vi "main(test).vi"() -> ()   [LabVIEW 2020]
uses:
  stany.ctl
  <vilib>/Analysis/1siggen.llb/Ramp Pattern by Samples.vi
  <vilib>/Utility/file.llb/Write Delimited Spreadsheet (DBL).vi
  lib/VirtualLab.lvlibp/VISASimulator/VISALib.lvlib
  lib/VirtualLab.lvlibp/Devices/Devices.lvlib
  lib/VirtualLab.lvlibp/Models/Exercise.lvlib
  <vilib>/Analysis/NI_AALBase.lvlib
panel:
  in  "Samples":i32=800
  out "Error":bool
  out "Error source":string
  in  "Save":bool
  out "Connection HP_dvm1":bool
  out "Actual Power [mW]":dbl
  in  "Pmax [mW]":dbl=200.0
  in  "Ib[uA]":dbl(ring) items=["0"=0.0, "100"=0.0001, "200"=0.0002, "300"=0.0003, "400"=0.0004]
  out "Ic=f(Uce)":cluster{dbl[], "Ramp Pattern":dbl[]}(graph)
  out "Ic[A]":dbl
  out "Uce [V]":dbl
  in  "Cancel Button":bool
  out "Progres":u8(slide) scale=0.0..100.0
  in  "stop/resume":bool
  in  "Measure":bool
  in  "Connect":bool
  out "Connection HP_zas":bool
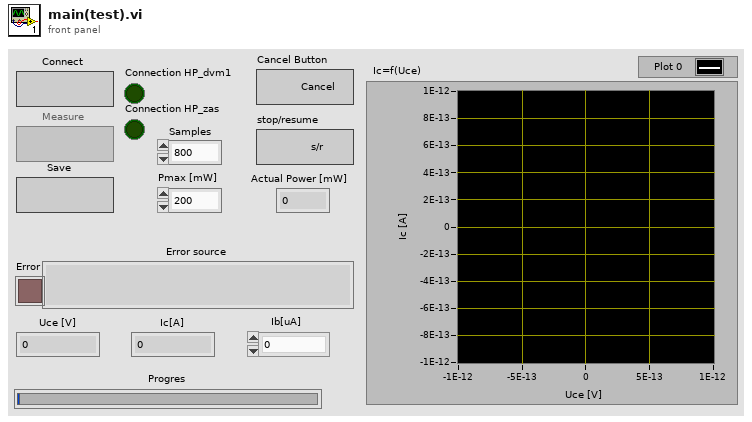
[diagram p1: front panel]
types:
  T1 = cluster{"HP_zas (PSU reference)":refnum<visa-resource-name>, "PSU_connecton":bool, "Ic":dbl[], "Uce":dbl[], "HP_dvm1(DMM reference)":refnum<visa-resource-name>, "DMM_connecton":bool}
  T2 = typedef "stany.ctl" = enum16{"init", "wait", "connect", "measure", "end", "save", "error"}
  T3 = enum8{"Enabled", "Disabled", "Disabled and Grayed Out"}
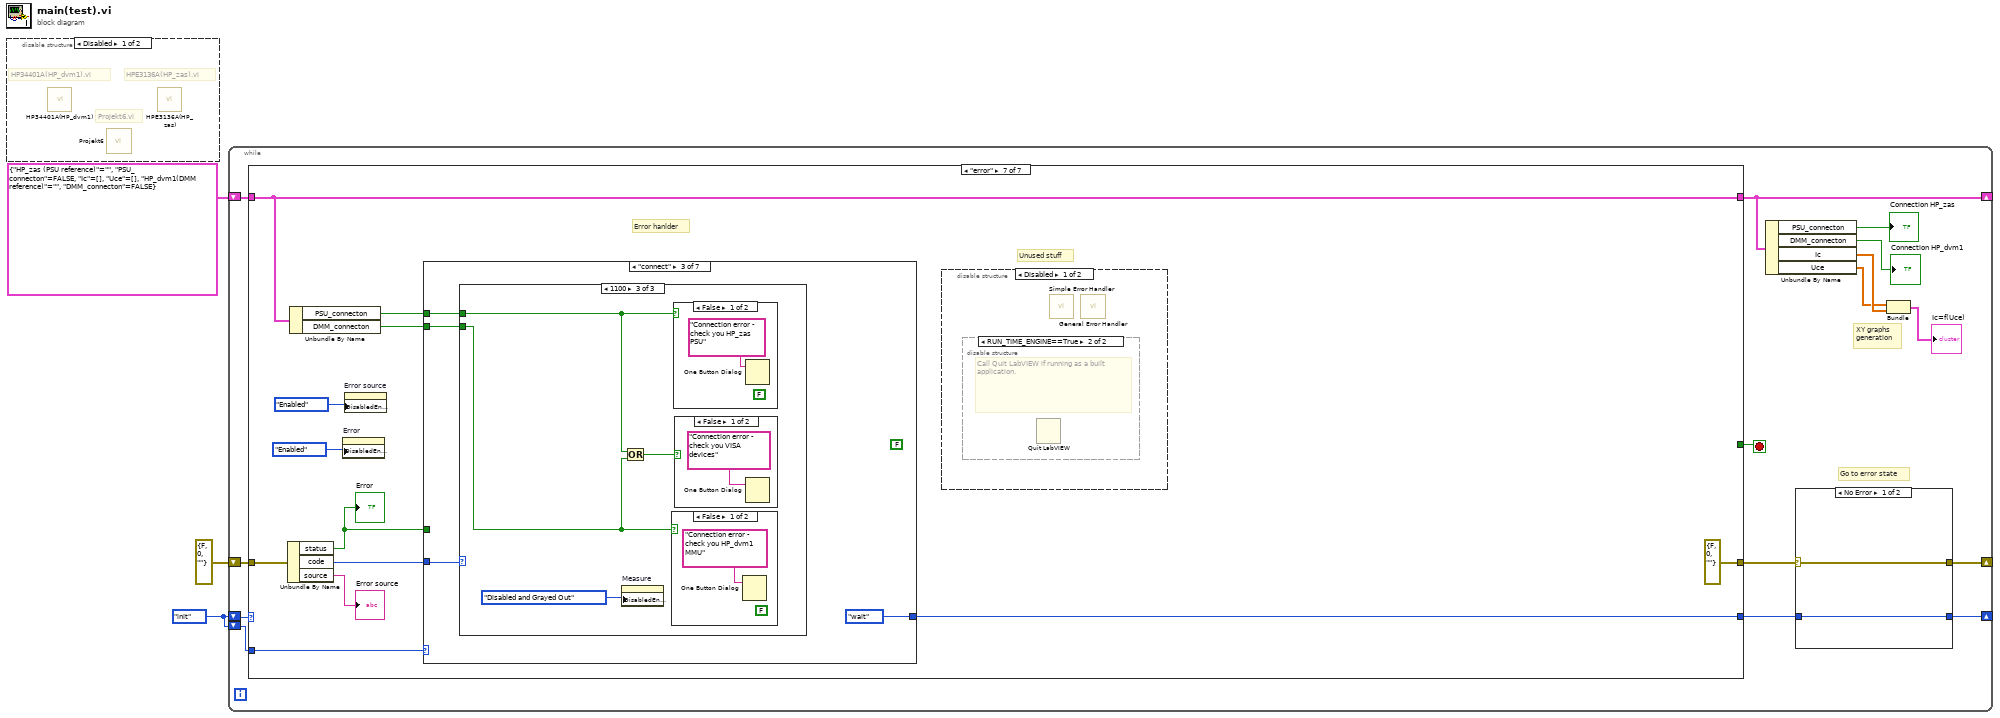
[diagram p0: block diagram]
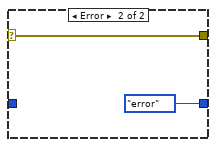
[diagram p3: hidden frame]
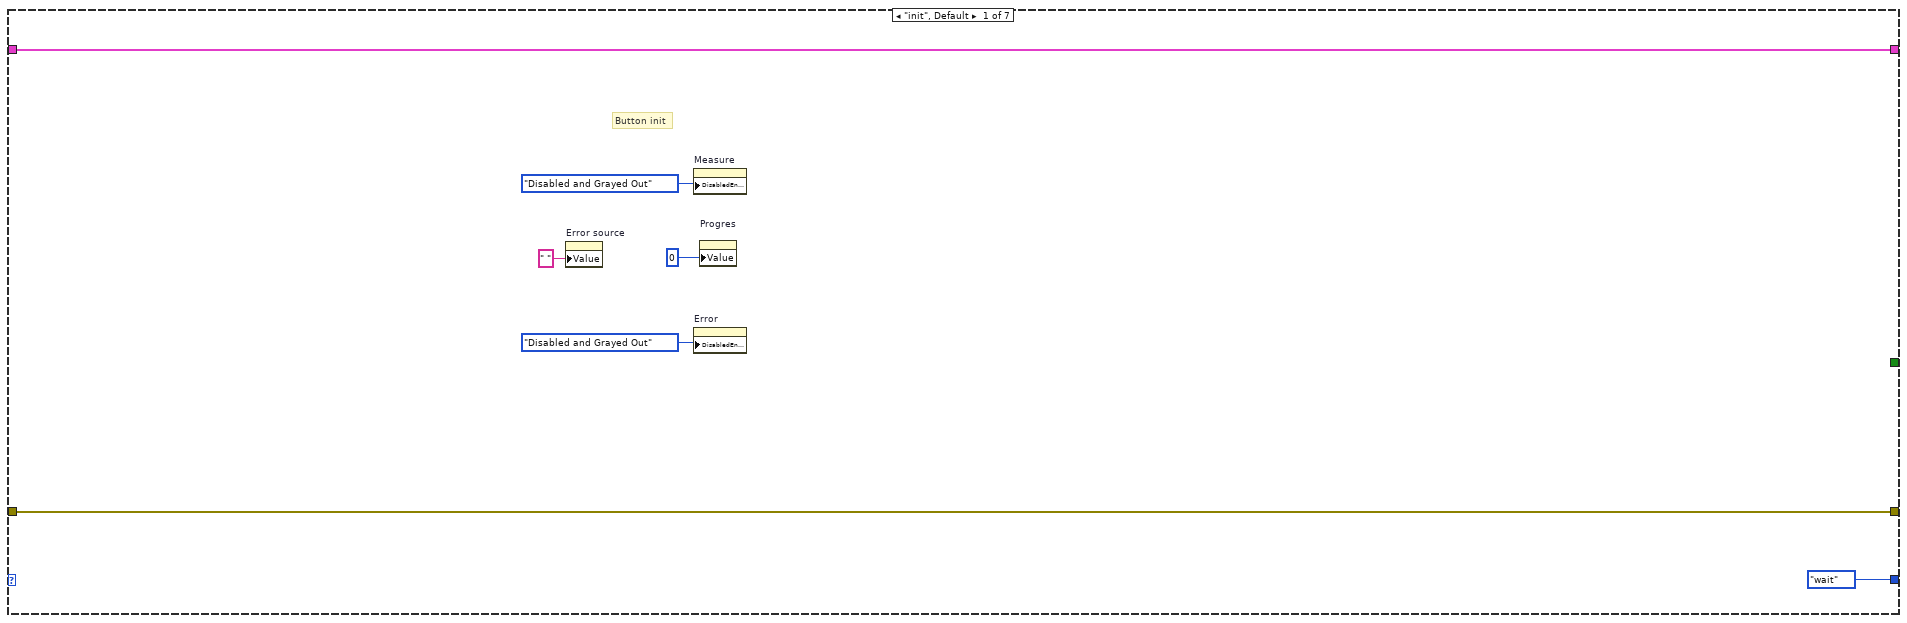
[diagram p4: hidden frame]
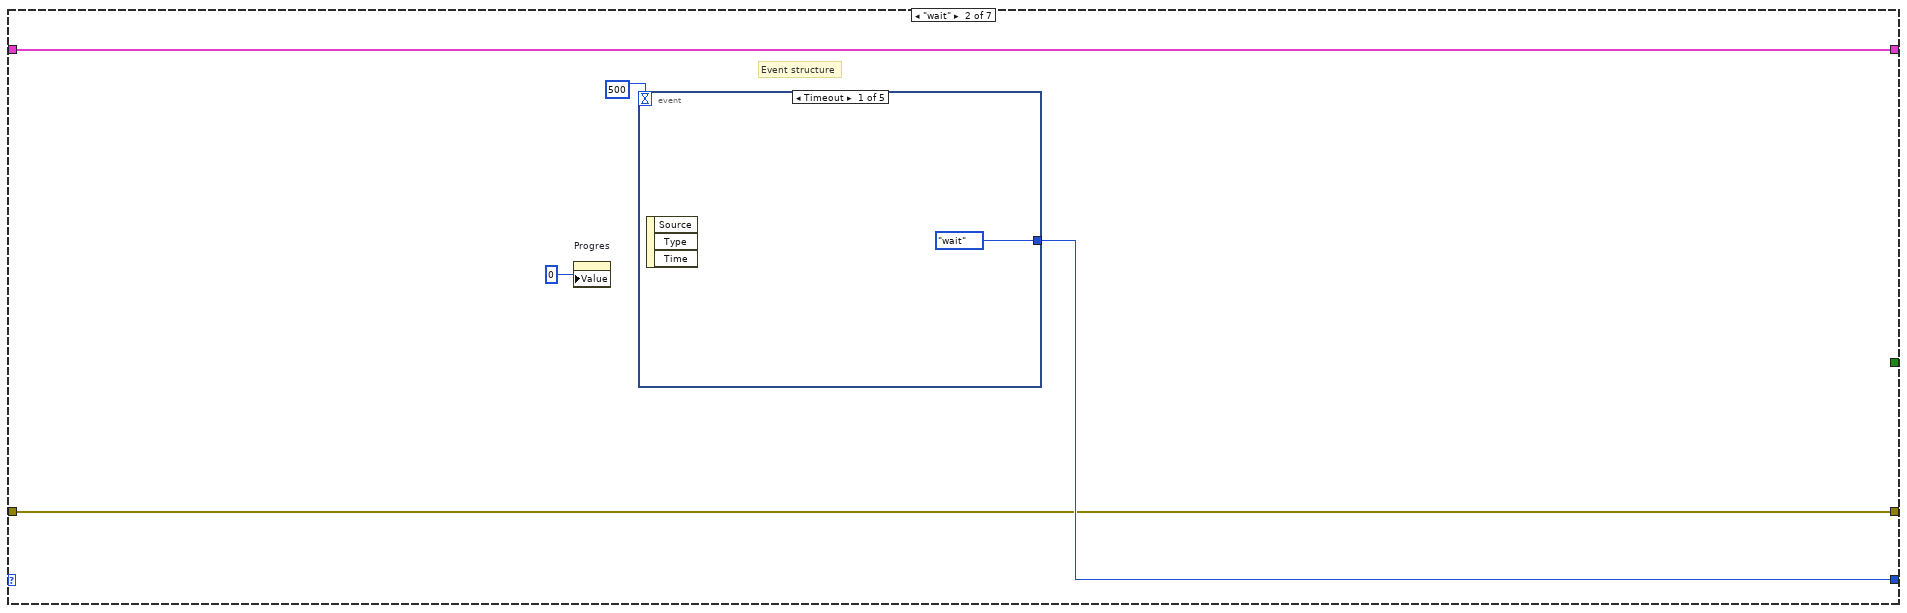
[diagram p5: hidden frame]
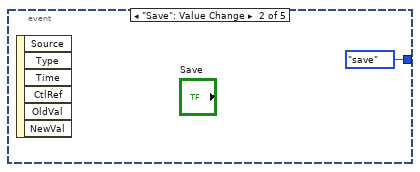
[diagram p6: hidden frame]
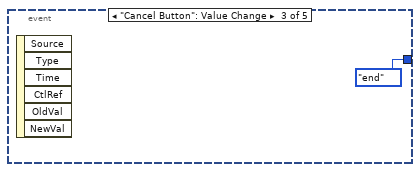
[diagram p7: hidden frame]
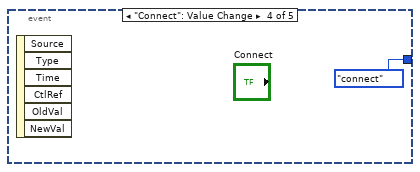
[diagram p8: hidden frame]
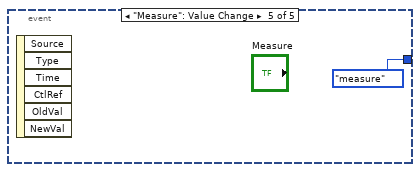
[diagram p9: hidden frame]
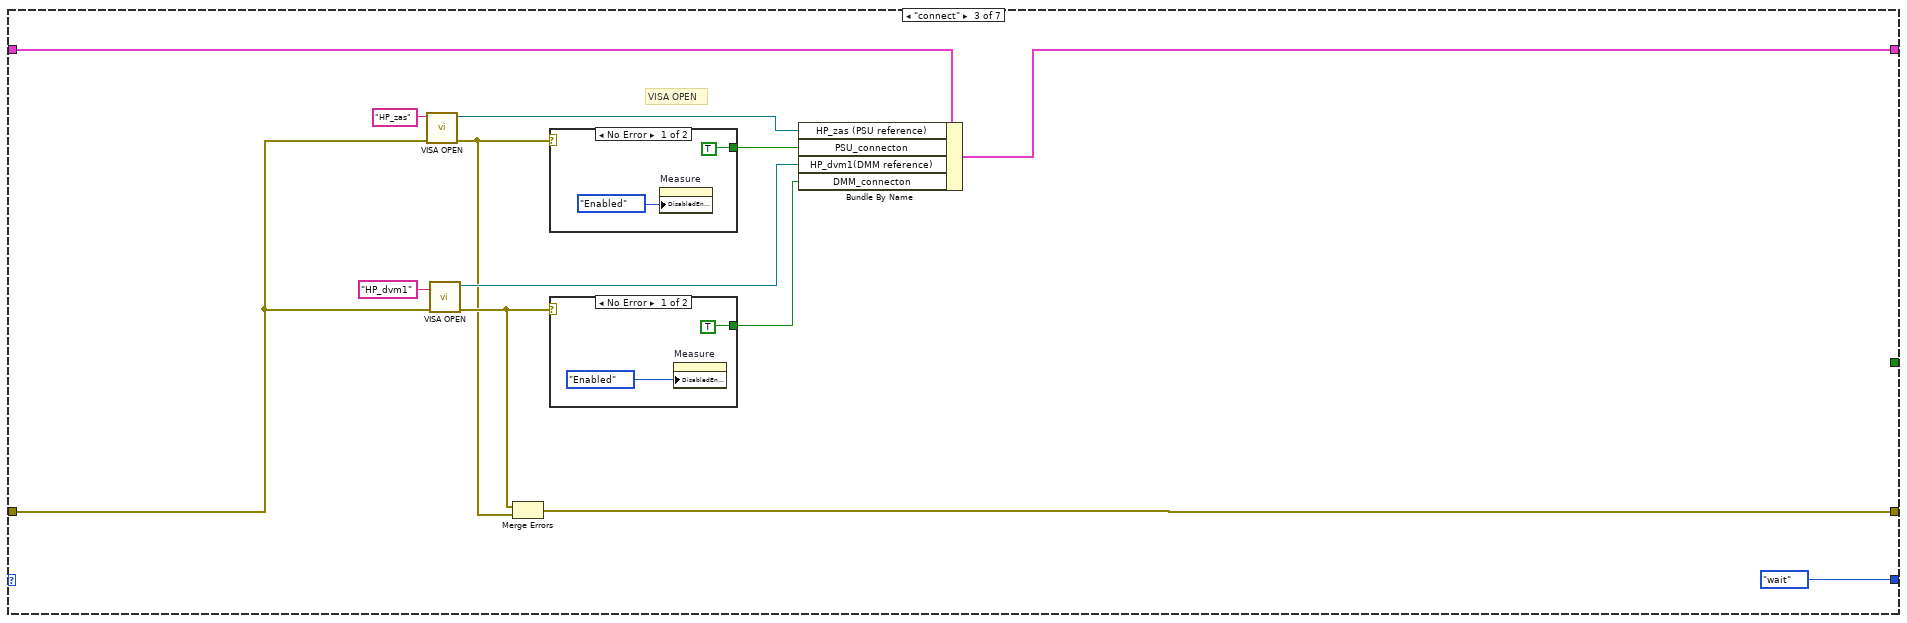
[diagram p10: hidden frame]
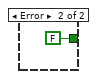
[diagram p11: hidden frame]
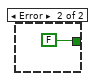
[diagram p12: hidden frame]
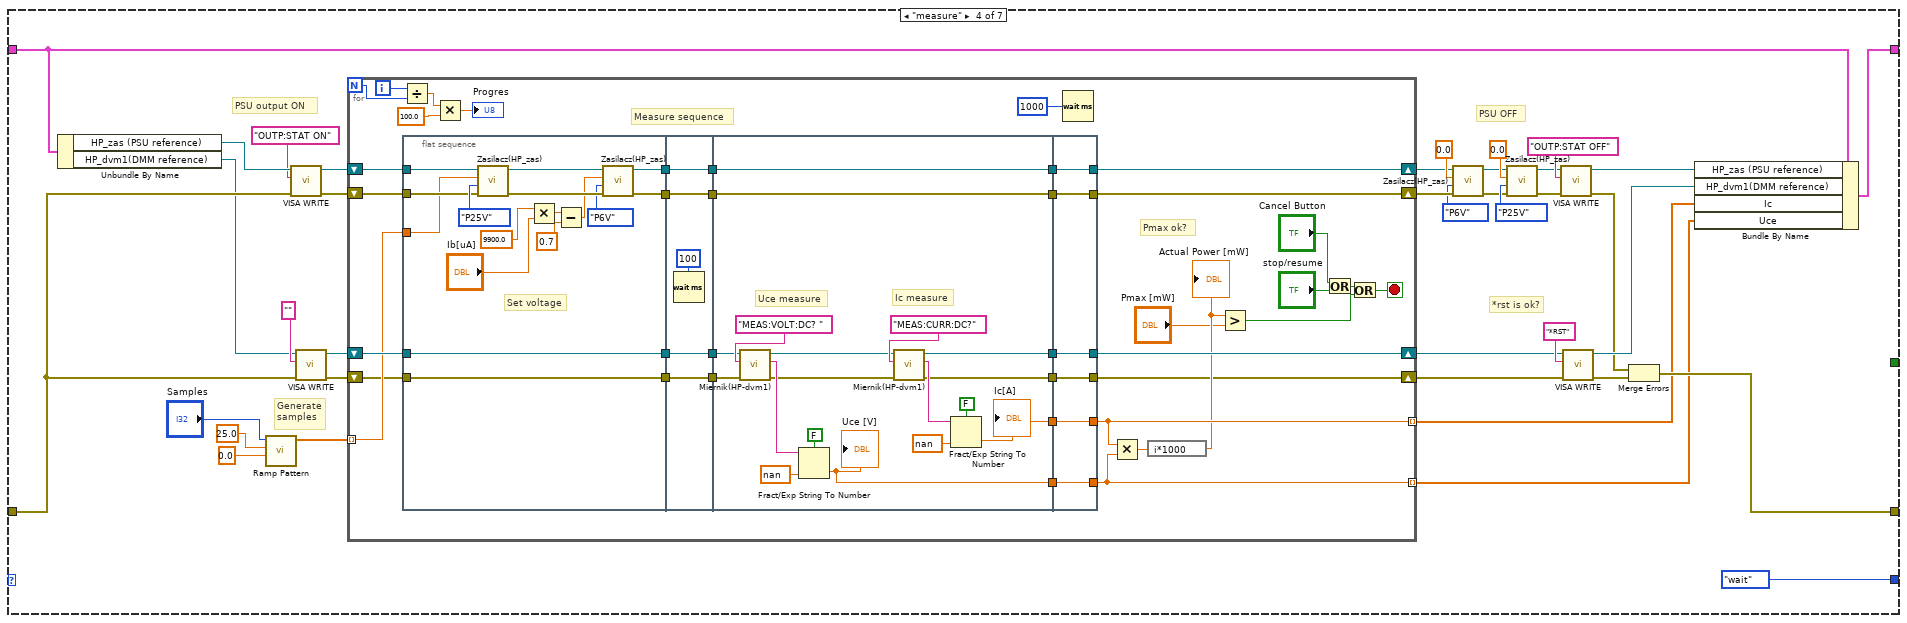
[diagram p13: hidden frame]
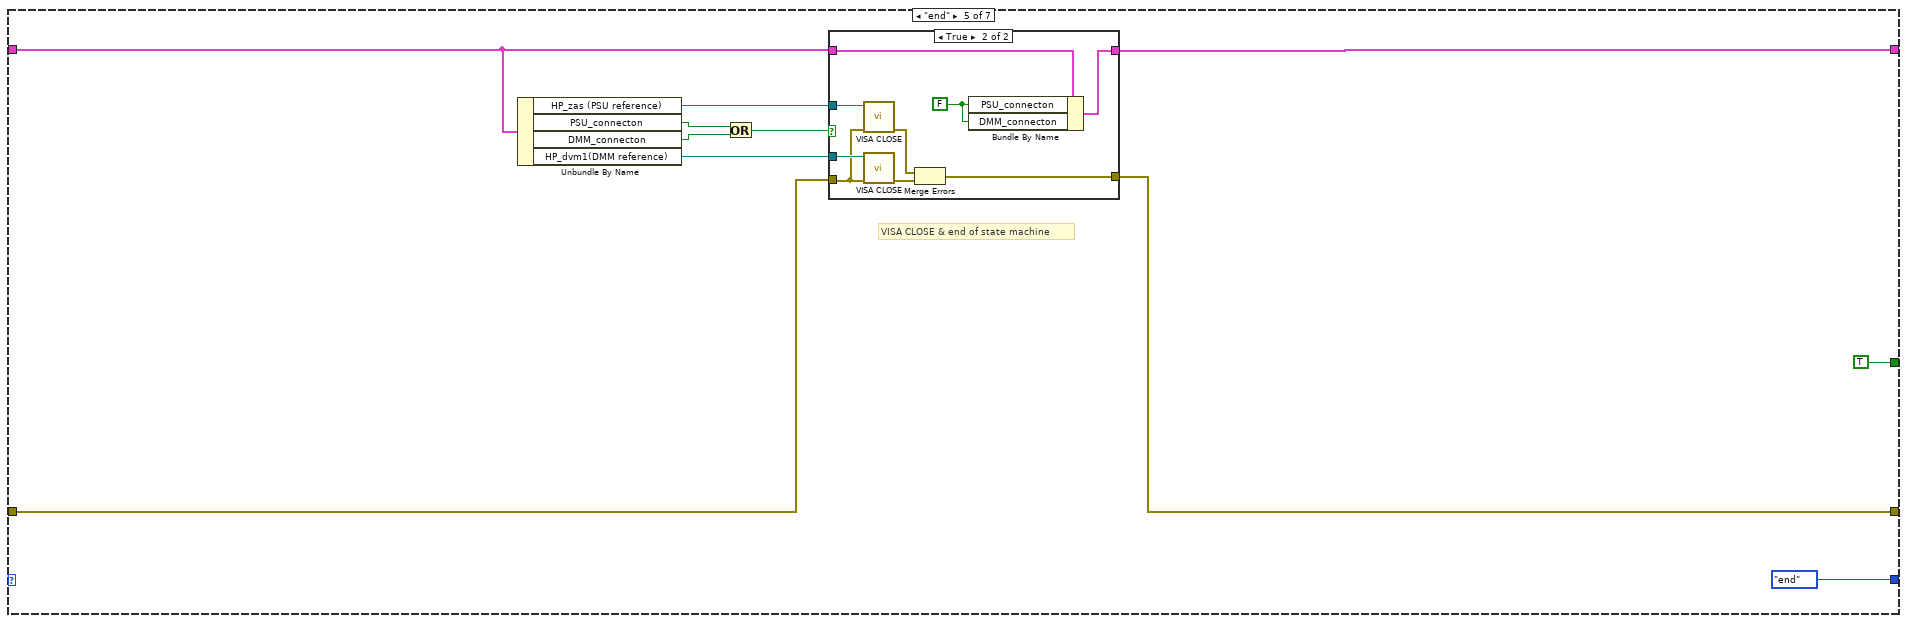
[diagram p14: hidden frame]
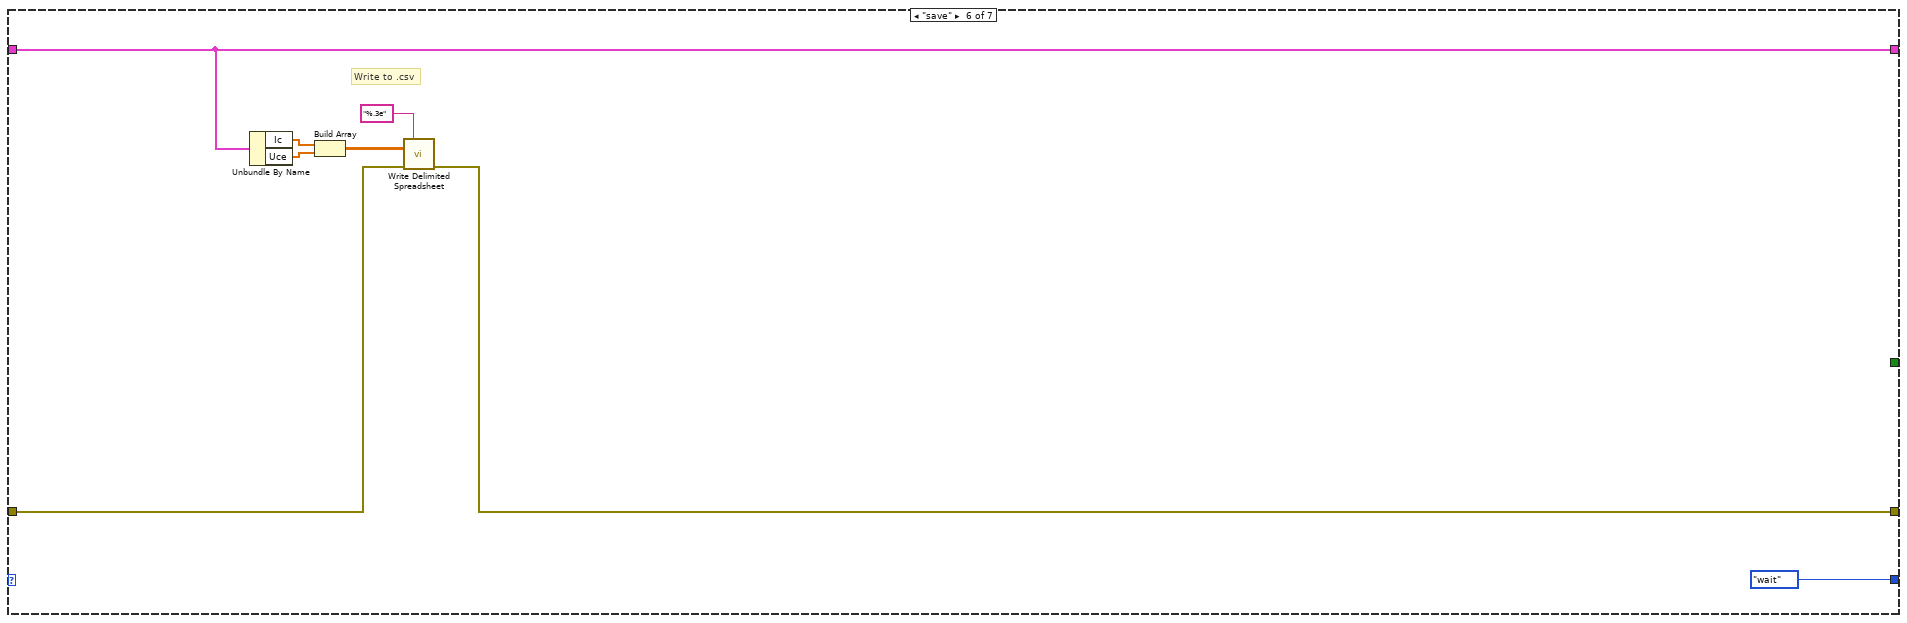
[diagram p16: hidden frame]
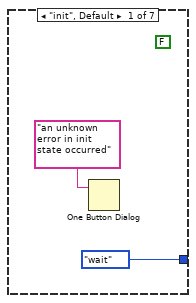
[diagram p19: hidden frame]
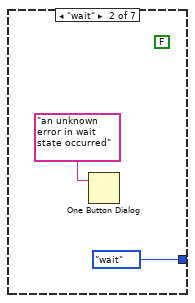
[diagram p20: hidden frame]
diagram:
  w1 = stany."init"
  n1 = disable-structure shown="Disabled" {
    frame Disabled {
      # "Projekt6.vi"
      # "HPE3136A(HP_zas).vi"
      # "HP34401A(HP_dvm1).vi"
      n2 = call "HP34401A(HP_dvm1).vi"() -> ()  [unwired: 12 in]
      n3 = call "Projekt6.vi"() -> ()  [unwired: 12 in]
      n4 = call "HPE3136A(HP_zas).vi"() -> ()  [unwired: 12 in]
    }
    frame Enabled {
    }
  }
  n5 = while {
    shift-right: [w10] -> _
    shift-left: w1 -> [w18]
    shift-right: [w9] -> _
    shift-left: T1 {"HP_zas (PSU reference)"="", "PSU_connecton"=FALSE, "Ic"=[], "Uce"=[], "HP_dvm1(DMM reference)"="", "DMM_connecton"=FALSE} -> [w16]
    shift-right: [w12] -> _
    shift-left: errorcluster {"status"=FALSE, "code"=0, "source"=""} ("error constant") -> [w14]
    shift-left: w1 -> [w7]
    stop <- w17 stop-if-true
    # "Go to error state"
    # "XY graphs\ngeneration"
    n6 = case shown="\"error\"" w18 {
      tunnel: [stany."wait" w33 stany."wait" stany."wait" stany."end" stany."wait" w215] -> w11
      tunnel: [_ _ _ _ TRUE _ _] -> w17
      tunnel: w16 -> [w27 w32 w46 w78 w186 w208 w212]
      tunnel: [w27 w32 w48 w94 w187 w208 w212] -> w9
      tunnel: w14 -> [w25 w30 w40 w76 w181 w202 w219]
      tunnel: [w25 w30 w43 w73 w180 w203 errorcluster {"status"=FALSE, "code"=0, "source"=""} ("error out")] -> w13
      tunnel: w7 -> [_ _ _ _ _ _ w220]
      frame "init", Default {
        # "Button init"
        n7 = property on="Error source" class="Str"("Value"=" " ("Error source")) -> ()  [unwired: 2 in, 2 out]
        n8 = property on="Measure" class="Bool"("DisabledEnum"=T3."Disabled and Grayed Out" ("Disabled")) -> ()  [unwired: 2 in, 2 out]
        n9 = property on="Error" class="Bool (strict)"("DisabledEnum"=T3."Disabled and Grayed Out" ("Disabled")) -> ()  [unwired: 2 in, 2 out]
        n10 = property on="Progres" class="Slide (strict)"("Value"=u8 0 ("Progres")) -> ()  [unwired: 2 in, 2 out]
      }
      frame "wait" {
        # "Event structure"
        n11 = property on="Progres" class="Slide (strict)"("Value"=u8 0 ("Progres")) -> ()  [unwired: 2 in, 2 out]
        n12 = event shown="[0] Timeout" {
          selector: _ -> [_ _ _ _ _]
          dyn-events: _ -> [_ _ _ _ _]
          timeout: 500 -> [_ _ _ _ _]
          tunnel: [stany."wait" stany."save" stany."end" stany."connect" stany."measure"] -> w33
          event Timeout {
            n13 = event-data() -> ()  [unwired: 1 in, 3 out]
          }
          event "Save": Value Change {
            n14 = event-data() -> ()  [unwired: 1 in, 6 out]
          }
          event "Cancel Button": Value Change {
            n15 = event-data() -> ()  [unwired: 1 in, 6 out]
          }
          event "Connect": Value Change {
            n16 = event-data() -> ()  [unwired: 1 in, 6 out]
          }
          event "Measure": Value Change {
            n17 = event-data() -> ()  [unwired: 1 in, 6 out]
          }
        }
      }
      frame "connect" {
        # "VISA OPEN"
        n18 = call "VISA OPEN.vi"("error in (no error)"=w40, "VISA resource name"="HP_zas") -> ("error out"=w41:errorcluster, "VISA resource name out"=w51:refnum<visa-resource-name>)  [unwired: 8 in]
        n19 = call "VISA OPEN.vi"("error in (no error)"=w40, "VISA resource name"="HP_dvm1") -> ("error out"=w42:errorcluster, "VISA resource name out"=w45:refnum<visa-resource-name>)  [unwired: 8 in]
        n20 = Merge Errors(w42, w41) -> (w43:errorcluster)
        n21 = case shown="No Error" w41 {
          tunnel: [TRUE FALSE ("connecton")] -> w50
          frame No Error {
            n22 = property on="Measure" class="Bool"("DisabledEnum"=T3."Enabled" ("Disabled")) -> ()  [unwired: 2 in, 2 out]
          }
          frame Error {
          }
        }
        n23 = case shown="No Error" w42 {
          tunnel: [TRUE FALSE ("connecton")] -> w44
          frame No Error {
            n24 = property on="Measure" class="Bool"("DisabledEnum"=T3."Enabled" ("Disabled")) -> ()  [unwired: 2 in, 2 out]
          }
          frame Error {
          }
        }
        n25 = Bundle By Name(cluster=w46, "HP_zas (PSU reference)"=w51, "PSU_connecton"=w50, "HP_dvm1(DMM reference)"=w45, "DMM_connecton"=w44) -> (w48:T1)
      }
      frame "measure" {
        # "PSU output ON"
        # "Generate\nsamples"
        # "*rst is ok?"
        # "PSU OFF"
        n26 = Unbundle By Name(w78) -> ("HP_zas (PSU reference)"=w70:refnum<visa-resource-name>, "HP_dvm1(DMM reference)"=w59:refnum<visa-resource-name>)
        n27 = call-poly <vilib>:"Ramp Pattern.vi"("start"=0.0, "end"=25.0, "samples"="Samples") -> ("Ramp Pattern"=w63:dbl[])  [unwired: 7 in, 1 out]
        n28 = call "VISA WRITE.vi"("error in (no error)"=w76, "write buffer"="OUTP:STAT ON" ("format string"), "VISA resource name"=w70) -> ("error out"=w64:errorcluster, "VISA resource name out"=w67:refnum<visa-resource-name>)  [unwired: 6 in, 1 out]
        n29 = call "VISA WRITE.vi"("error in (no error)"=w76, "write buffer"="" ("format string"), "VISA resource name"=w59) -> ("error out"=w61:errorcluster, "VISA resource name out"=w62:refnum<visa-resource-name>)  [unwired: 6 in, 1 out]
        n30 = for {
          N -> [w127]
          shift-right: [w123] -> w84
          shift-left: w67 -> [w115]
          tunnel: [w107] -> w71 mode=indexing
          shift-right: [w122] -> w83
          shift-left: w64 -> [w114]
          tunnel: w63 -> [w110] mode=indexing
          tunnel: [w108] -> w72 mode=indexing
          shift-right: [w120] -> w80
          shift-left: w62 -> [w111]
          shift-right: [w100] -> w79
          shift-left: w61 -> [w98]
          i -> [w128]
          stop <- w101 stop-if-true
          # "Pmax ok?"
          # "Measure sequence"
          n31 = Divide(x=w128, y=w127) -> (x/y=w133:dbl)
          n32 = flat-sequence {
            tunnel: [w143] -> w118
            tunnel: [w144] -> w116
            tunnel: w115 -> [w149]
            tunnel: w114 -> [w148]
            tunnel: [w147] -> w112
            tunnel: w111 -> [w147]
            tunnel: w110 -> [w141]
            tunnel: w98 -> [w135]
            tunnel: [w135] -> w97
            tunnel: [w154] -> w119
            tunnel: w118 -> [w154]
            tunnel: [w153] -> w117
            tunnel: w116 -> [w153]
            tunnel: [w152] -> w113
            tunnel: w112 -> [w152]
            tunnel: w97 -> [w151]
            tunnel: [w151] -> w96
            tunnel: [w167] -> w126
            tunnel: [w168] -> w125
            tunnel: [w169] -> w124
            tunnel: [w159] -> w121
            tunnel: w119 -> [w168]
            tunnel: w117 -> [w167]
            tunnel: w113 -> [w166]
            tunnel: [w158] -> w109
            tunnel: [w157] -> w99
            tunnel: w96 -> [w156]
            tunnel: w126 -> [w178]
            tunnel: w125 -> [w177]
            tunnel: w124 -> [w179]
            tunnel: [w179] -> w107
            tunnel: [w178] -> w123
            tunnel: [w177] -> w122
            tunnel: w121 -> [w176]
            tunnel: [w176] -> w120
            tunnel: w109 -> [w175]
            tunnel: [w175] -> w108
            tunnel: [w174] -> w100
            tunnel: w99 -> [w174]
            frame #0 {
              # "Set voltage"
              n33 = call "Zasilacz(HP_zas).vi"("error in (no error)"=w148, "Source"=enum16{"P6V", "P25V"}."P25V" ("Kanal"), "Voltage"=w141, "VISA Refnum in"=w149) -> ("error out"=w145:errorcluster, "VISA Refnum out"=w146:refnum<visa-resource-name>)  [unwired: 6 in]
              n34 = Multiply(x=9900.0, y="Ib[uA]") -> (x*y=w138:dbl)
              n35 = Subtract(x=w138, y=0.7) -> (x-y=w140:dbl)
              n36 = call "Zasilacz(HP_zas).vi"("error in (no error)"=w145, "Source"=enum16{"P6V", "P25V"}."P6V" ("Kanal"), "Voltage"=w140, "VISA Refnum in"=w146) -> ("error out"=w143:errorcluster, "VISA Refnum out"=w144:refnum<visa-resource-name>)  [unwired: 6 in]
            }
            frame #1 {
              n37 = Wait (ms)(milliseconds to wait=u32 100) -> ()  [unwired: 1 out]
            }
            frame #2 {
              # "Ic measure"
              # "Uce measure"
              n38 = call "Miernik(HP-dvm1).vi"("error in (no error)"=w156, "write buffer"="MEAS:VOLT:DC? ", "VISA Refnum in"=w166) -> ("error out"=w161:errorcluster, "read buffer"=w173:string, "VISA Refnum out"=w160:refnum<visa-resource-name>)  [unwired: 6 in]
              n39 = Fract/Exp String To Number(use system decimal point (T)=FALSE, string=w173, default (0 dbl)=nan) -> (number=w169:dbl)  [unwired: 1 in, 1 out]
              "Uce [V]" <- w169
              n40 = call "Miernik(HP-dvm1).vi"("error in (no error)"=w161, "write buffer"="MEAS:CURR:DC?", "VISA Refnum in"=w160) -> ("error out"=w157:errorcluster, "read buffer"=w165:string, "VISA Refnum out"=w159:refnum<visa-resource-name>)  [unwired: 6 in]
              n41 = Fract/Exp String To Number(use system decimal point (T)=FALSE, string=w165, default (0 dbl)=nan) -> (number=w158:dbl)  [unwired: 1 in, 1 out]
              "Ic[A]" <- w158
            }
            frame #3 {
            }
          }
          n42 = Multiply(x=w133, y=100.0) -> (x*y=→"Progres":dbl)
          n43 = Wait (ms)(milliseconds to wait=u32 1000) -> ()  [unwired: 1 out]
          n44 = Multiply(x=w108, y=w107) -> (x*y=w106:dbl)
          n45 = expression code="i*1000"(w106) -> (w105:dbl)
          "Actual Power [mW]" <- w105
          n46 = Greater?(x=w105, y="Pmax [mW]") -> (0:w102:bool)
          n47 = Or(x="Cancel Button", y="stop/resume") -> (x .or. y?=w103:bool)
          n48 = Or(x=w103, y=w102) -> (x .or. y?=w101:bool)
        }
        n49 = call "Zasilacz(HP_zas).vi"("error in (no error)"=w83, "Source"=enum16{"P6V", "P25V"}."P6V" ("Kanal"), "Voltage"=0.0 ("Napiecie 2"), "VISA Refnum in"=w84) -> ("error out"=w86:errorcluster, "VISA Refnum out"=w85:refnum<visa-resource-name>)  [unwired: 6 in]
        n50 = call "Zasilacz(HP_zas).vi"("error in (no error)"=w86, "Source"=enum16{"P6V", "P25V"}."P25V" ("Kanal"), "Voltage"=0.0 ("Napiecie 2"), "VISA Refnum in"=w85) -> ("error out"=w88:errorcluster, "VISA Refnum out"=w89:refnum<visa-resource-name>)  [unwired: 6 in]
        n51 = call "VISA WRITE.vi"("error in (no error)"=w88, "write buffer"="OUTP:STAT OFF" ("format string"), "VISA resource name"=w89) -> ("error out"=w75:errorcluster, "VISA resource name out"=w93:refnum<visa-resource-name>)  [unwired: 6 in, 1 out]
        n52 = call "VISA WRITE.vi"("error in (no error)"=w79, "write buffer"="*RST" ("format string"), "VISA resource name"=w80) -> ("error out"=w74:errorcluster, "VISA resource name out"=w77:refnum<visa-resource-name>)  [unwired: 6 in, 1 out]
        n53 = Merge Errors(w75, w74) -> (w73:errorcluster)
        n54 = Bundle By Name(cluster=w78, "HP_zas (PSU reference)"=w93, "HP_dvm1(DMM reference)"=w77, "Ic"=w72, "Uce"=w71) -> (w94:T1)
      }
      frame "end" {
        # "VISA CLOSE & end of state machine"
        n55 = Unbundle By Name(w186) -> ("HP_zas (PSU reference)"=w188:refnum<visa-resource-name>, "PSU_connecton"=w184:bool, "DMM_connecton"=w183:bool, "HP_dvm1(DMM reference)"=w185:refnum<visa-resource-name>)
        n56 = Or(x=w184, y=w183) -> (x .or. y?=w182:bool)
        n57 = case shown="True" w182 {
          tunnel: w188 -> [_ w201]
          tunnel: w186 -> [w192 w200]
          tunnel: [w192 w198] -> w187
          tunnel: w185 -> [_ w197]
          tunnel: [w191 w194] -> w180
          tunnel: w181 -> [w191 w195]
          frame False {
          }
          frame True {
            w199 = FALSE ("connecton")
            n58 = call "VISA CLOSE.vi"("error in (no error)"=w195, "VISA resource name"=w201) -> ("error out"=w193:errorcluster)  [unwired: 9 in]
            n59 = call "VISA CLOSE.vi"("error in (no error)"=w195, "VISA resource name"=w197) -> ("error out"=w196:errorcluster)  [unwired: 9 in]
            n60 = Merge Errors(w193, w196) -> (w194:errorcluster)
            n61 = Bundle By Name(cluster=w200, "PSU_connecton"=w199, "DMM_connecton"=w199) -> (w198:T1)
          }
        }
      }
      frame "save" {
        # "Write to .csv"
        n62 = Unbundle By Name(w208) -> ("Ic"=w207:dbl[], "Uce"=w206:dbl[])
        n63 = Build Array(w207, w206) -> (w205:dbl[][])
        n64 = call-poly <vilib>:"Write Delimited Spreadsheet.vi"("format (%.3f)"="%.3e", "2D data"=w205, "error in (no error)"=w202) -> ("error out"=w203:errorcluster)  [unwired: 11 in, 1 out]
      }
      frame "error" {
        # "Unused stuff"
        # "Error hanlder"
        n65 = Unbundle By Name(w219) -> ("status"=w217:bool, "code"=w218:i32, "source"=→"Error source":string)
        "Error" <- w217
        n66 = Unbundle By Name(w212) -> ("PSU_connecton"=w211:bool, "DMM_connecton"=w210:bool)
        n67 = property on="Error" class="Bool (strict)"("DisabledEnum"=T3."Enabled" ("Disabled")) -> ()  [unwired: 2 in, 2 out]
        n68 = property on="Error source" class="Str"("DisabledEnum"=T3."Enabled" ("Disabled")) -> ()  [unwired: 2 in, 2 out]
        n69 = case shown="\"connect\"" w220 {
          tunnel: w218 -> [_ _ w229 _ _ _ _]
          tunnel: w217 -> [_ _ _ _ _ _ _]
          tunnel: [stany."wait" stany."wait" stany."wait" stany."wait" stany."wait" stany."wait" stany."wait"] -> w215
          tunnel: w211 -> [_ _ w227 _ _ _ _]
          tunnel: w210 -> [_ _ w226 _ _ _ _]
          frame "init", Default {
            (unwired) FALSE ("status")
            n70 = One Button Dialog(message="an unknown error in init state occurred") -> ()  [unwired: 1 in, 1 out]
          }
          frame "wait" {
            (unwired) FALSE ("status")
            n71 = One Button Dialog(message="an unknown error in wait state occurred") -> ()  [unwired: 1 in, 1 out]
          }
          frame "connect" {
            (unwired) FALSE ("status")
            n72 = case shown="1100" w229 {
              tunnel: w227 -> [_ _ w233]
              tunnel: w226 -> [_ _ w232]
              frame 0, Default {
              }
              frame 1 {
                n73 = One Button Dialog(message="an unknown error in connect state occurred") -> ()  [unwired: 1 in, 1 out]
              }
              frame 1100 {
                n74 = property on="Measure" class="Bool"("DisabledEnum"=T3."Disabled and Grayed Out" ("Disabled")) -> ()  [unwired: 2 in, 2 out]
                n75 = Or(x=w233, y=w232) -> (x .or. y?=w234:bool)
                n76 = case shown="False" w232 {
                  frame False {
                    (unwired) FALSE ("connecton")
                    n77 = One Button Dialog(message="Connection error - check you HP_dvm1 MMU") -> ()  [unwired: 1 in, 1 out]
                  }
                  frame True {
                  }
                }
                n78 = case shown="False" w233 {
                  frame False {
                    (unwired) FALSE ("connecton")
                    n79 = One Button Dialog(message="Connection error - check you HP_zas PSU") -> ()  [unwired: 1 in, 1 out]
                  }
                  frame True {
                  }
                }
                n80 = case shown="False" w234 {
                  frame False {
                    n81 = One Button Dialog(message="Connection error - check you VISA devices") -> ()  [unwired: 1 in, 1 out]
                  }
                  frame True {
                  }
                }
              }
            }
          }
          frame "measure" {
            (unwired) FALSE ("status")
            n82 = One Button Dialog(message="an unknown error in measure state occurred") -> ()  [unwired: 1 in, 1 out]
          }
          frame "end" {
            (unwired) FALSE ("status")
            n83 = One Button Dialog(message="an unknown error in end state  occurred") -> ()  [unwired: 1 in, 1 out]
          }
          frame "save" {
            (unwired) FALSE ("status")
            n84 = One Button Dialog(message="an unknown errorin save state occurred") -> ()  [unwired: 1 in, 1 out]
          }
          frame "error" {
            (unwired) FALSE ("status")
            n85 = One Button Dialog(message="an unknown error occurred") -> ()  [unwired: 1 in, 1 out]
          }
        }
        n86 = disable-structure shown="Disabled" {
          frame Disabled {
            n87 = disable-structure shown="RUN_TIME_ENGINE==True" {
              frame condition #0 (active) {
              }
              frame condition #1 {
                # "Call Quit LabVIEW if running as a built application."
                n88 = Quit LabVIEW() -> ()  [unwired: 1 in]
              }
            }
            n89 = call <vilib>:"Simple Error Handler.vi"() -> ()  [unwired: 5 in, 5 out]
            n90 = call <vilib>:"General Error Handler.vi"() -> ()  [unwired: 11 in, 5 out]
          }
          frame Enabled {
          }
        }
      }
    }
    n91 = Unbundle By Name(w9) -> ("PSU_connecton"=→"Connection HP_zas":bool, "DMM_connecton"=→"Connection HP_dvm1":bool, "Ic"=w6:dbl[], "Uce"=w5:dbl[])
    n92 = case shown="No Error" w13 {
      selector: w13 -> [w20 w21]
      tunnel: [w20 w21] -> w12
      tunnel: w11 -> [w19 _]
      tunnel: [w19 stany."error"] -> w10
      frame No Error {
      }
      frame Error {
      }
    }
    n93 = Bundle("Uce"=w5, "Ic"=w6) -> (→"Ic=f(Uce)":cluster{"Uce":dbl[], "Ic":dbl[]})  [unwired: 1 in]
  }
